vi "Edit Data.vi"(8 "error in (no error)":errorcluster, 10 "All Data":refnum<class "Data Item.lvclass">[](array[class]), 11 "Element in":refnum<class "Element.lvclass">) -> (0 "error out":errorcluster, 1 "OK?":bool, 2 "All Data out":refnum<class "Data Item.lvclass">[](array[class]), 3 "Element out":refnum<class "Element.lvclass">)   [LabVIEW 2026, in "VILab.lvlib" / "Element.lvclass"]
uses:
  Element.lvclass
  Data Item/Data Item.lvclass
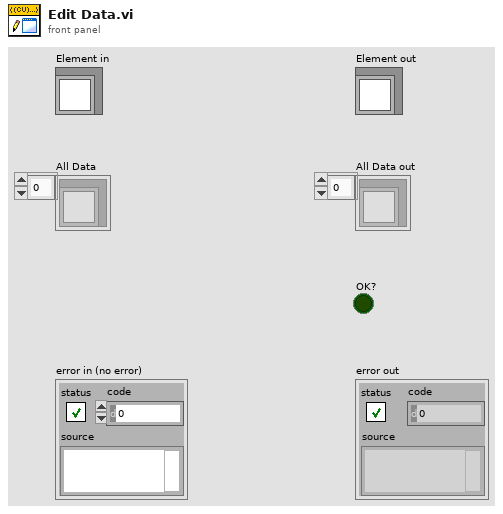
[diagram p1: front panel]
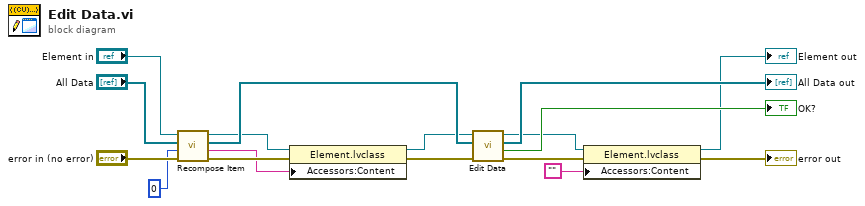
[diagram p0: block diagram]
diagram:
  n1 = call-dynamic "Recompose Item.vi"("error in (no error)"="error in (no error)", "Nesting Level"=0, "All Data"="All Data", "Element in"="Element in") -> ("error out"=w13:errorcluster, "XML String"=w7:string, "All Data out"=w9:refnum<class "Data Item.lvclass">[], "Element out"=w8:refnum<class "Element.lvclass">)  [unwired: 4 in]
  n2 = property class="Element.lvclass"(reference=w8, error in=w13, "Accessors:Content"=w7) -> (reference out=w6:refnum<class "Element.lvclass">, error out=w10:errorcluster)
  n3 = call-parent "Edit Data.vi"("error in (no error)"=w10, "All Data"=w9, "Data Item in"=w6) -> ("error out"=w17:errorcluster, "OK?"=→"OK?":bool, "All Data out"=→"All Data out":refnum<class "Data Item.lvclass">[], "Data Item out"=w3:refnum<class "Element.lvclass">)  [unwired: 5 in]
  n4 = property class="Element.lvclass"(reference=w3, error in=w17, "Accessors:Content"="") -> (reference out=→"Element out":refnum<class "Element.lvclass">, error out=→"error out":errorcluster)
